vi "J1939 Claim Polymorphic.vi"   [LabVIEW 2015, in "J1939 runtime.lvclass"]
uses:
  J1939 runtime.lvclass
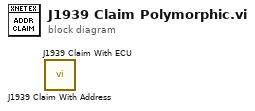
[diagram p0: block diagram]
diagram:
  n1 = call "J1939 Claim With Address.vi"() -> ()  [unwired: 9 in, 3 out]
  n2 = call "J1939 Claim With ECU.vi"() -> ()  [unwired: 9 in, 3 out]
